vi "NagleDemo-MessageReflector.vi"() -> ()   [LabVIEW 2012]
panel:
  out "value":i32
  in  "port":u16=5678
  out "error out":errorcluster
  # "This VI demonstrates the effect of having the TCP Nagle algorithm enabled or disabled on  a socket for a particular kind of query/response protocol.\n\nTo run this demo, first run this VI, then run its partner in crime,\nNagleDemo-MessageSender.vi, on another machine."
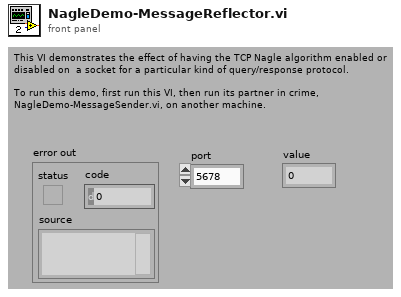
[diagram p1: front panel]
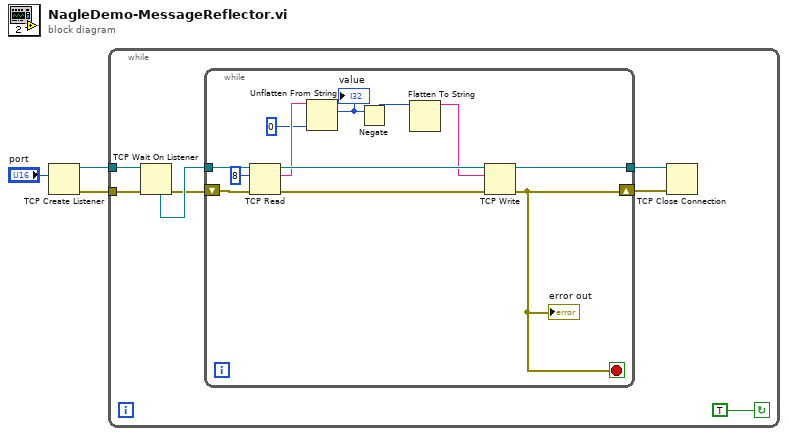
[diagram p0: block diagram]
diagram:
  n1 = TCP Create Listener(10:"port") -> (0:w2:errorcluster, 3:w3:refnum<k5>)  [unwired: 4 in, 1 out]
  n2 = while {
    tunnel: w3 -> [w10]
    tunnel: w2 -> [w7]
    stop <- TRUE continue-if-true
    n3 = TCP Wait On Listener(8:w7, 11:w10) -> (0:w6:errorcluster, 4:w9:refnum<k5>)  [unwired: 2 in, 3 out]
    n4 = while {
      tunnel: w9 -> [w22]
      tunnel: [w20] -> w8
      shift-right: [w11] -> w5
      shift-left: w6 -> [w12]
      stop <- w11 stop-if-true
      n5 = TCP Read(connection ID=w22, bytes to read=8, error in (no error)=w12) -> (connection ID out=w21:refnum<k5>, data out=w18:string, error out=w13:errorcluster)  [unwired: 2 in]
      n6 = Unflatten From String(type=0, binary string=w18) -> (value=w16:i32)  [unwired: 3 in, 2 out]
      "value" <- w16
      n7 = Negate(x=w16) -> (-x=w15:i32)
      n8 = Flatten To String(anything=w15) -> (data string=w14:string)  [unwired: 3 in, 2 out]
      n9 = TCP Write(connection ID=w21, data in=w14, error in (no error)=w13) -> (connection ID out=w20:refnum<k5>, error out=w11:errorcluster)  [unwired: 1 in, 1 out]
      "error out" <- w11
    }
    n10 = TCP Close Connection(connection ID=w8, error in (no error)=w5) -> ()  [unwired: 1 in, 2 out]
  }
